vi "Manual SetCurrent.vi"() -> ()   [LabVIEW 2024]
panel:
  in  "Current":dbl
  in  "Source":T1(ring)
  in  "stop":bool
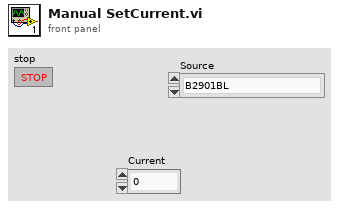
[diagram p1: front panel]
types:
  T1 = enum16{"B2901BL", "USB-3104 10M o/p3", "USB-3104 100K o/p5"}
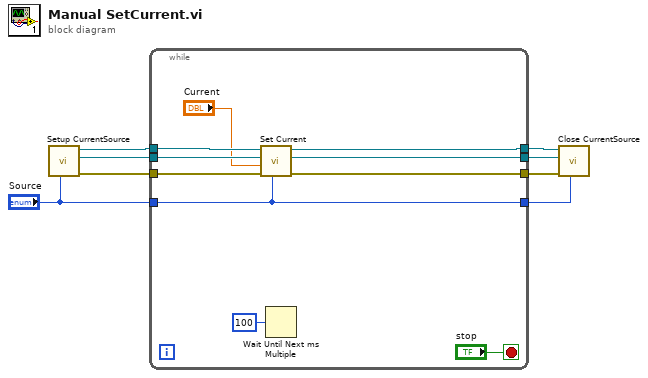
[diagram p0: block diagram]
diagram:
  n1 = call "Setup CurrentSource.vi"("Source"="Source") -> ("error out"=w8:errorcluster, "task out"=w6:refnum<k24>, "VISA Refnum out"=w4:refnum<visa-resource-name>)  [unwired: 8 in]
  n2 = while {
    tunnel: w8 -> [w17]
    tunnel: [w16] -> w7
    tunnel: w6 -> [w15]
    tunnel: [w14] -> w5
    tunnel: w4 -> [w13]
    tunnel: [w12] -> w3
    tunnel: [w11] -> w1
    tunnel: "Source" -> [w11]
    stop <- "stop" stop-if-true
    n3 = call "Set Current.vi"("Source 2"=w11, "error in (no error)"=w17, "Current"="Current", "task in"=w15, "VISA Refnum in"=w13) -> ("error out"=w16:errorcluster, "task out"=w14:refnum<k24>, "VISA Refnum out"=w12:refnum<visa-resource-name>)  [unwired: 4 in]
    n4 = Wait Until Next ms Multiple(millisecond multiple=u32 100) -> ()  [unwired: 1 out]
  }
  n5 = call "Close CurrentSource.vi"("Source 2"=w1, "error in (no error)"=w7, "task in"=w5, "VISA Refnum in"=w3) -> ()  [unwired: 8 in]
